vi "AlarmDataToTimestamp.vi"(8 "Error In":errorcluster, 10 "Coords":T1, 11 "CtlRef":refnum<vi>) -> (0 "error out":errorcluster, 2 "XY":cluster{"X":dbl, "Y":dbl}, 3 "min index(es)":i32)   [LabVIEW 2018]
doc: "Convert mouse click coordinates to X, Y values (which are the amplitude and timestamp values of the waveforms in the graph)."
uses:
  <vilib>/Utility/miscctls.llb/LVPoint32TypeDef.ctl
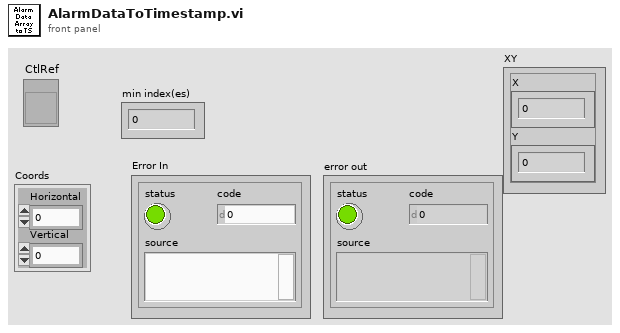
[diagram p1: front panel]
types:
  T1 = typedef "LVPoint32TypeDef.ctl" = cluster{"Horizontal":i32, "Vertical":i32}
  T2 = typedef "LVRectTypeDef.ctl" = cluster{"Left":i16, "Top":i16, "Right":i16, "Bottom":i16}
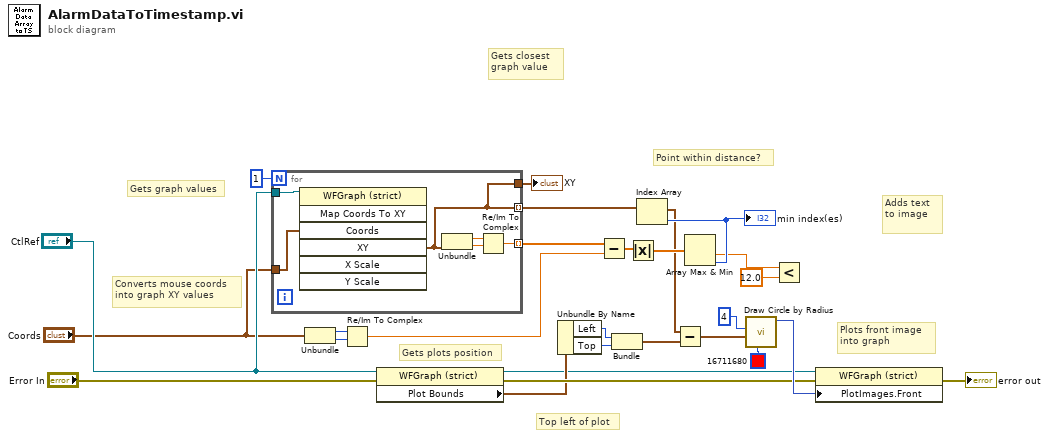
[diagram p0: block diagram]
diagram:
  # "Point within distance?"
  # "Gets closest graph value"
  # "Gets graph values"
  # "Gets plots position"
  # "Top left of plot"
  # "Adds text to image"
  # "Plots front image \ninto graph"
  # "Converts mouse coords\ninto graph XY values"
  n1 = for {
    N: 1 -> [_]
    tunnel: [w31] -> w21 mode=indexing
    tunnel: "CtlRef" -> [w30]
    tunnel: [w28] -> w7 mode=indexing
    tunnel: "Coords" -> [w29]
    tunnel: [w28] -> w1
    n2 = invoke on="Invoke Node" class="WFGraph (strict)" method="Map Coords To XY"(reference=w30, "Coords"=w29) -> ("XY"=w28:cluster{"X":dbl, "Y":dbl})  [unwired: 5 in, 6 out]
    n3 = Unbundle(w28) -> ("X"=w33:dbl, "Y"=w32:dbl)
    n4 = Re/Im To Complex(1:w32, 2:w33) -> (0:w31:cdb)
  }
  "XY" <- w1
  n5 = Unbundle("Coords") -> ("Horizontal"=w23:i32, "Vertical"=w22:i32)
  n6 = Re/Im To Complex(1:w22, 2:w23) -> (0:w20:cdb)
  n7 = property on="Property Node" class="WFGraph (strict)"(reference="CtlRef", error in="Error In") -> (reference out=w8:refnum<vi>, error out=w24:errorcluster, "Plot Bounds"=w15:T2)
  n8 = Unbundle By Name(w15) -> ("Left"=w14:i16, "Top"=w13:i16)
  n9 = Subtract(x=w21, y=w20) -> (x-y=w19:cdb[])
  n10 = Bundle("Left"=w14, "Top"=w13) -> (w12:cluster{"Left":i16, "Top":i16})  [unwired: 1 in]
  n11 = Absolute Value(x=w19) -> (abs(x)=w18:dbl[])
  n12 = Array Max & Min(array=w18) -> (min value=w16:dbl, min index (indices)=w17:i32)  [unwired: 2 out]
  "min index(es)" <- w17
  n13 = Index Array(array=w7, index=w17) -> (element=w9:cluster{"X":dbl, "Y":dbl})
  n14 = Subtract(x=w9, y=w12) -> (x-y=w11:cluster{dbl, dbl})
  n15 = call <vilib>:"Draw Circle by Radius.vi"("color(black)"=u32 16711680 ("text color(black)"), "pixel center"=w11, "radius"=i16 4) -> ("new picture"=w25:picture)  [unwired: 8 in]
  n16 = Less?(x=w16, y=12.0 ("x")) -> ()  [unwired: 1 out]
  n17 = property on="Property Node" class="WFGraph (strict)"(reference=w8, error in=w24, "PlotImages.Front"=w25) -> (error out=→"error out":errorcluster)  [unwired: 1 out]
